vi "FT-IR Background Diagnose.vi"   [LabVIEW 2020, in "FT-IR.lvlib"]
uses:
  FT-IR.lvlib
  FGV FT-IR Diagnose Aktionen.ctl
  SysLog/SysLog Interface.ctl
  SysLog/SysLog.lvlib
panel:
  # "FTIR Diagnose bei Kalibrieren aufzeichnen"
types:
  T1 = typedef "SysLog.lvlib/SysLog Interface.ctl" = cluster{"FehlermeldungsCode":i32, "ErfolgsmeldungsCode":i32, "ParameterListenString":string, "Anzeige":bool, "SysLogIcon":enum16{"OK", "Warnung", "Fehler"}, "intern":bool}
  T2 = typedef "FT-IR.lvlib/FGV FT-IR Diagnose Aktionen.ctl" = enum16{"Lesen", "Diagnose Schreiben", "Min Schreiben", "Max Schreiben"}
  T3 = typedef "FT-IR.lvlib/TOOLweb Interface.lvlib/Typdefinitionen.lvlib/TOOLweb Diagnose.ctl" = cluster{"(14) temperature":sgl, "(15) pressure":sgl, "(16) oxygen":sgl, "(50) diag-igramdc":sgl, "(51) diag-igrampp":sgl, "(52) diag-phaseAngle":sgl, "(53) diag-laserpp":sgl, "(54) diag-laserdc":sgl, "(55) diag-badscan":sgl, "(56) diag-centerburst":sgl, "(57) diag-linearizerCheck":sgl, "(58) diag-SNR":sgl, "(59) diag-sBeamIntensity":sgl}
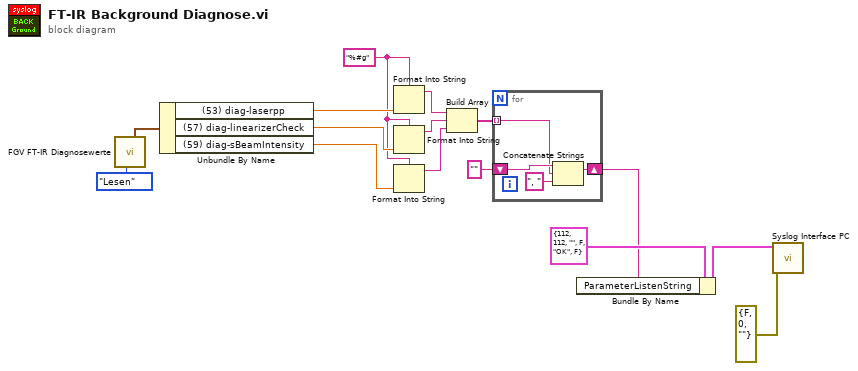
[diagram p0: block diagram]
diagram:
  w12 = "%#g" ("Format-String")
  n1 = call "FGV FT-IR Diagnosewerte.vi"("Aktionen"=FGV_FT-IR_Diagnose_Aktionen."Lesen") -> ("Diagnose"=w10:T3)  [unwired: 5 in, 5 out]
  n2 = Unbundle By Name(w10) -> ("(53) diag-laserpp"=w13:sgl, "(57) diag-linearizerCheck"=w14:sgl, "(59) diag-sBeamIntensity"=w15:sgl)
  n3 = Format Into String(format string=w12, w13) -> (resulting string=w6:string)  [unwired: 2 in, 1 out]
  n4 = Format Into String(format string=w12, w14) -> (resulting string=w5:string)  [unwired: 2 in, 1 out]
  n5 = Format Into String(format string=w12, w15) -> (resulting string=w4:string)  [unwired: 2 in, 1 out]
  n6 = Build Array(w6, w5, w4) -> (w3:string[])
  n7 = for {
    tunnel: w3 -> [w16] mode=indexing
    shift-right: [w18] -> w1
    shift-left: "" -> [w19]
    n8 = Concatenate Strings(w19, w16, ", " ("String")) -> (w18:string)
  }
  n9 = Bundle By Name(cluster=T1 {"FehlermeldungsCode"=112, "ErfolgsmeldungsCode"=112, "ParameterListenString"="", "Anzeige"=FALSE, "SysLogIcon"=enum."OK", "intern"=FALSE} ("Cluster (in)"), "ParameterListenString"=w1) -> (w7:T1)
  n10 = call "Syslog Interface PC.vi"("Fehler (in)"=errorcluster {"status"=FALSE, "code"=0, "source"=""}, "Cluster (in)"=w7) -> ()  [unwired: 9 in, 1 out]
